vi "Sort 2D String Array - String or Number.vi"(7 "Input String (\" \")":string) -> (8 "Is Num? (F)":bool)   [LabVIEW 2010, in "xijk_select_best_filter.lvlib"]
doc: "Sort 2D String Array - String or Number.vi\n\n<B>Description:</B>\n\nThis VI scans the input string and outputs a boolean True if all characters in the input string are digits ranging from 0 through 9, A through F, or a through f. The characters .,+ and - are ignored. \n\n<B>Usage:</B>\n\nWire all required inputs.\n\n<B>Inputs:</B>\n\nInput String\n- The string to scan.\n\n<B>Outputs:</B>\n\nIs Num? (F)\n- This boolean is set True if the input string represents a number.\n\n<B>Developed by:</B>\n\nMark Ridgley\nmark.ridgley@logicpd.com"
uses:
  xijk_select_best_filter.lvlib
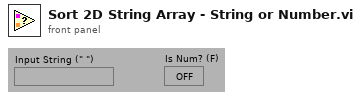
[diagram p1: front panel]
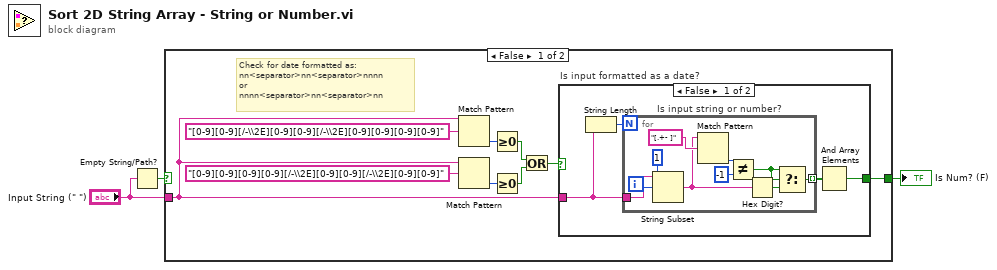
[diagram p0: block diagram]
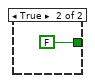
[diagram p2: hidden frame]
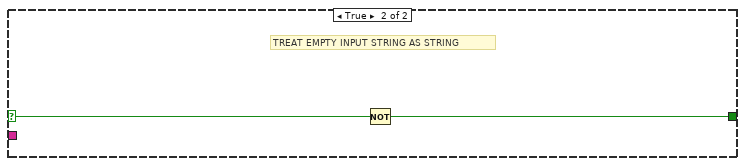
[diagram p3: hidden frame]
diagram:
  n1 = Empty String/Path?(string/path="Input String (\" \")") -> (empty?=w1:bool)
  n2 = case shown="False" w1 {
    selector: w1 -> [_ w29]
    tunnel: "Input String (\" \")" -> [w7 _]
    tunnel: [w12 w28] -> w3
    frame False {
      # "Check for date formatted as:\nnn<separator>nn<separator>nnnn\nor\nnnnn<separator>nn<separator>nn"
      n3 = Match Pattern(string=w7, regular expression="[0-9][0-9][/-\\2E][0-9][0-9][/-\\2E][0-9][0-9][0-9][0-9]") -> (offset past match=w8:i32)  [unwired: 4 out]
      n4 = Match Pattern(string=w7, regular expression="[0-9][0-9][0-9][0-9][/-\\2E][0-9][0-9][/-\\2E][0-9][0-9]") -> (offset past match=w11:i32)  [unwired: 4 out]
      n5 = Greater Or Equal To 0?(x=w8) -> (x >= 0?=w5:bool)
      n6 = Greater Or Equal To 0?(x=w11) -> (x >= 0?=w6:bool)
      n7 = Or(x=w5, y=w6) -> (x .or. y?=w4:bool)
      n8 = case "Is input formatted as a date?" shown="False" w4 {
        tunnel: w7 -> [w16 _]
        tunnel: [w15 FALSE] -> w12
        frame False {
          n9 = String Length(string=w16) -> (length=w13:i32)
          n10 = for "Is input string or number?" {
            N: w13 -> [_]
            tunnel: w16 -> [w22]
            tunnel: [w21] -> w14 mode=indexing
            i -> [w26]
            n11 = String Subset(string=w22, offset (0)=w26, length (rest)=1 ("length")) -> (substring=w19:string)
            n12 = Match Pattern(string=w19, regular expression="[.+- ]") -> (offset past match=w18:i32)  [unwired: 4 out]
            n13 = Not Equal?(x=w18, y=-1) -> (x != y?=w24:bool)
            n14 = Hex Digit?(1:w19) -> (0:w23:bool)
            n15 = Select(t=w24, s=w24, f=w23) -> (s? t:f=w21:bool)
          }
          n16 = And Array Elements(Boolean array=w14) -> (logical AND=w15:bool)
        }
        frame True {
        }
      }
    }
    frame True {
      # "TREAT EMPTY INPUT STRING AS STRING"
      n17 = Not(x=w29) -> (.not. x?=w28:bool)
    }
  }
  "Is Num? (F)" <- w3
